vi "FTW-Router-Construct.vi"(5 "Incoming Message Router Address":string="tcp://127.0.0.1:55555", 11 "error in":errorcluster) -> (4 "FTW Router":refnum<class "FTW-Router.lvclass">, 6 "Incoming Request":refnum<event-registration>, 8 "Inbox Address":string, 15 "error out":errorcluster)   [LabVIEW 2013, in "FTW-Actor.lvlib" / "FTW-Router.lvclass"]
uses:
  FTW-Router.lvclass
  Endpoint/FTW-Endpoint.lvclass
  FTW-Actor.lvlib
  Request/FTW-Request.lvclass
panel:
  # "Inputs"
  # "Outputs"
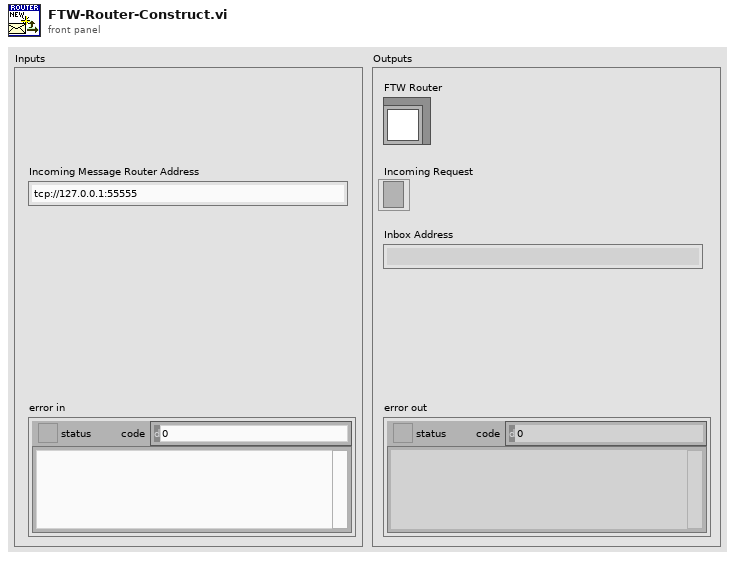
[diagram p1: front panel]
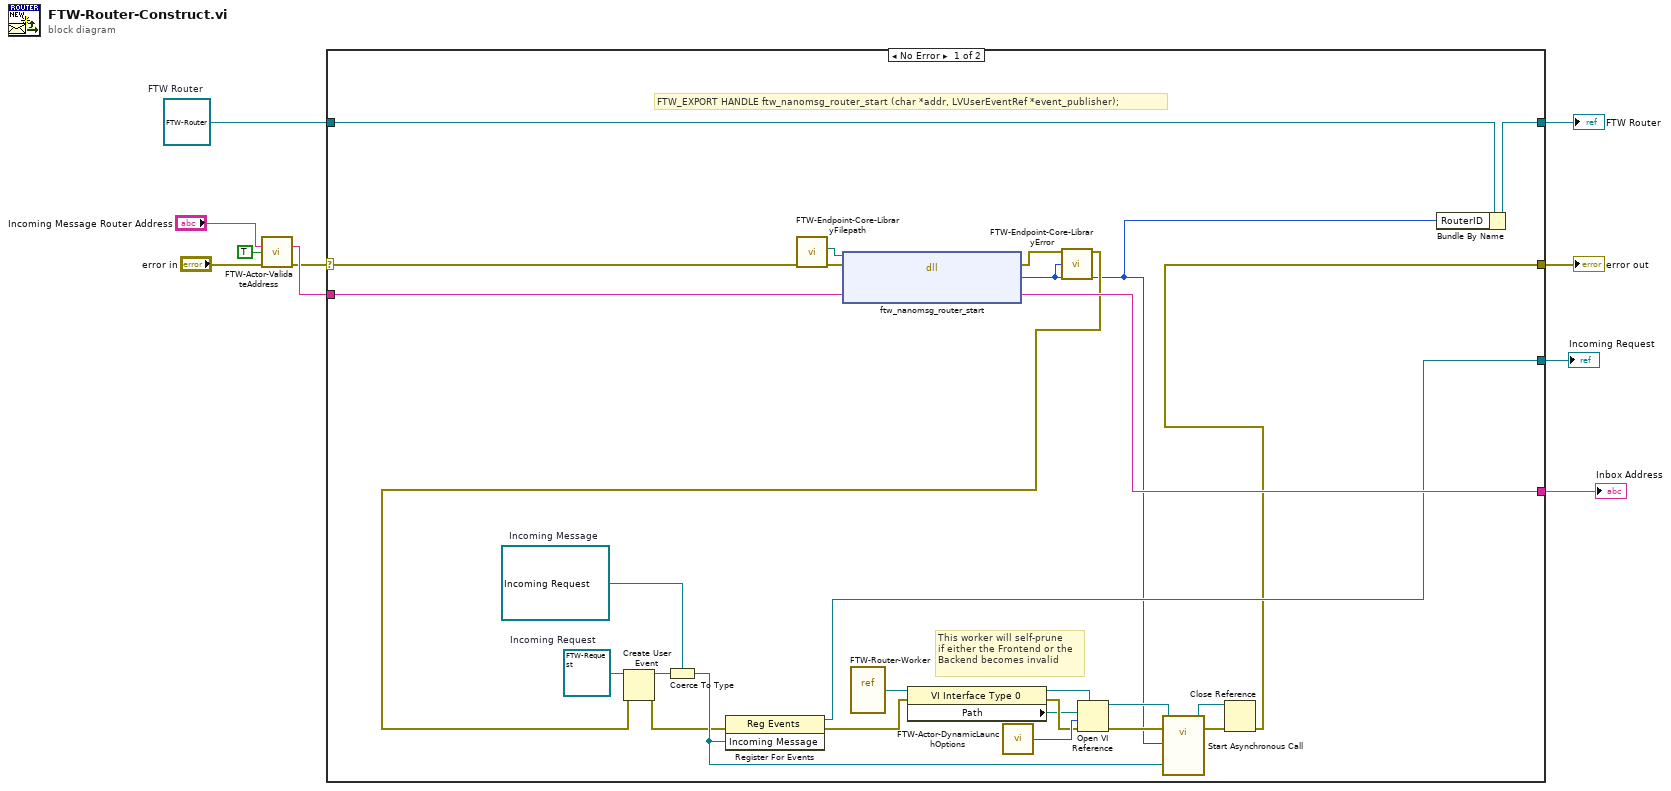
[diagram p0: block diagram]
diagram:
  w8 = refnum<class "FTW-Router.lvclass"> refnum  # FTW Router
  n1 = call "FTW-Actor-ValidateAddress.vi"("Address"="Incoming Message Router Address", "Allow wildcard replacement?"=TRUE, "error in"="error in") -> ("Sanitized Address"=w5:string, "error out"=w3:errorcluster)  [unwired: 10 in, 1 out]
  n2 = case shown="No Error" w3 {
    selector: w3 -> [w15 w39]
    tunnel: [w36 w38] -> w10
    tunnel: [w11 w39] -> w9
    tunnel: w8 -> [w37 w38]
    tunnel: w5 -> [w16 _]
    tunnel: [w20 _] -> w1
    tunnel: [w35 _] -> w7
    frame No Error {
      w19 = refnum<class "FTW-Request.lvclass"> refnum  # Incoming Request
      w30 = refnum<user-event> refnum  # Incoming Message
      # "This worker will self-prune\nif either the Frontend or the\nBackend becomes invalid"
      # "FTW_EXPORT HANDLE ftw_nanomsg_router_start (char *addr, LVUserEventRef *event_publisher);"
      n3 = call "FTW-Endpoint-Core-LibraryFilepath.vi"("error in"=w15) -> ("error out"=w17:errorcluster, "Library Filepath"=w18:path)  [unwired: 8 in, 1 out]
      n4 = dll-call lib="C:/Users/Jack/repo/ftw-master/Actor/src/Endpoint/Core/FTWLib-nanomsg32.dll" fn="ftw_nanomsg_router_start"(path in=w18, error in=w17, "Address"=w16) -> (error out=w14:errorcluster, "Return Value"=w12:i64, "Address"=w35:string)  [unwired: 1 in, 1 out]
      n5 = vi-ref "FTW-Router-Worker.vi"() -> (w21:refnum<vi>)
      n6 = call "FTW-Actor-DynamicLaunchOptions.vi"() -> ("Open VI Ref Options"=w26:i32)  [unwired: 1 in]
      n7 = call "FTW-Endpoint-Core-LibraryError.vi"("error in"=w14, "Return Value"=w12) -> ("error out"=w13:errorcluster)  [unwired: 13 in]
      n8 = Create User Event(user event datatype=w19, error in=w13) -> (user event=w29:refnum<user-event>, error out=w28:errorcluster)
      n9 = Coerce To Type(0:w29, 1:w30) -> (2:w34:refnum<user-event>)
      n10 = register-events(error in=w28, w34) -> (reference out=w20:refnum<event-registration>, error out=w31:errorcluster)  [unwired: 1 in]
      n11 = property class="VI Interface Type 0"(reference=w21, error in=w31) -> (reference out=w22:refnum<vi>, error out=w25:errorcluster, "Path"=w23:path)
      n12 = Open VI Reference(type specifier VI Refnum (for type only)=w22, vi path=w23, options=w26, error in (no error)=w25) -> (vi reference=w27:refnum<vi>, error out=w24:errorcluster)  [unwired: 2 in]
      n13 = call-by-ref "Start Asynchronous Call"(reference=w27, error in=w24, "Backend Handler"=w34, "RouterID"=w12) -> (reference out=w32:refnum<vi>, error out=w33:errorcluster)  [unwired: 1 in]
      n14 = Close Reference(reference=w32, error in (no error)=w33) -> (error out=w11:errorcluster)
      n15 = Bundle By Name(cluster=w37, "RouterID"=w12) -> (w36:refnum<class "FTW-Router.lvclass">)
    }
    frame Error {
    }
  }
  "error out" <- w9
  "FTW Router" <- w10
  "Inbox Address" <- w7
  "Incoming Request" <- w1
